vi "PulseFlash.vi"(4 "Time Target (ms)":i32=1) -> (1 "Flash":bool)   [LabVIEW 2017]
panel:
  out "OLD":u32
  out "NEW":u32
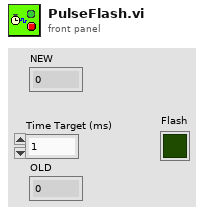
[diagram p1: front panel]
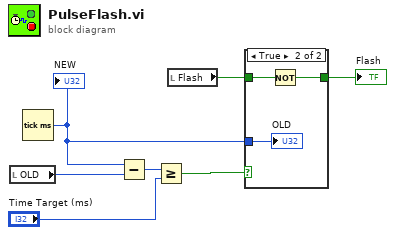
[diagram p0: block diagram]
diagram:
  n1 = local read "OLD"() -> (w5:u32)
  n2 = Tick Count (ms)() -> (millisecond timer value=w6:u32)
  "NEW" <- w6
  n3 = Subtract(x=w6, y=w5) -> (x-y=w3:u32)
  n4 = Greater Or Equal?(x=w3, y="Time Target (ms)") -> (x >= y?=w1:bool)
  n5 = local read "Flash"() -> (w4:bool)
  n6 = case shown="True" w1 {
    tunnel: [w8 w11] -> w7
    tunnel: w4 -> [w8 w10]
    tunnel: w6 -> [_ w9]
    frame False {
    }
    frame True {
      n7 = Not(x=w10) -> (.not. x?=w11:bool)
      "OLD" <- w9
    }
  }
  "Flash" <- w7
